vi "pre-processing.vi"() -> ()   [LabVIEW 2015]
uses:
  <vilib>/myRIO/Instrument Drivers/Onboard IO/AudioIn Block/typedefs/AudioIn Block Reference.ctl
  <vilib>/myRIO/Common/Instrument Driver Framework/Utilities/typedefs/myRIO Generic Hardware Reference.ctl
  <vilib>/myRIO/Common/Instrument Driver Framework/Utilities/typedefs/Hardware Version Enum.ctl
  <vilib>/myRIO/Common/Instrument Driver Framework/Utilities/typedefs/myRIO v1.0 Reference.ctl
  <vilib>/myRIO/Common/Instrument Driver Framework/Utilities/typedefs/Generic FPGA Reference.ctl
  <vilib>/myRIO/Common/Instrument Driver Framework/myRIO v1.0/AudioIn Block/typedefs/AudioIn Block Channels List.ctl
  <vilib>/myRIO/Common/Instrument Driver Framework/myRIO v1.0/AudioIn Block/typedefs/AudioIn Block Channels Enum.ctl
  <vilib>/myRIO/Common/Instrument Driver Framework/Utilities/typedefs/Analog Scaling Constants.ctl
  <vilib>/userdefined/High Color/nirio_resource_hc.ctl
  <vilib>/myRIO/Common/Instrument Driver Framework/Utilities/vis/Is FPGA Ref Available.vi
  <vilib>/myRIO/Common/Instrument Driver Framework/myRIO v1.0/AudioIn Block/vis/myRIO v1.1 Open Throughput AudioIn (N Samples).vi
  <vilib>/myRIO/Instrument Drivers/Onboard IO/AudioIn Block/vis/Read.vi
  <vilib>/myRIO/Common/Instrument Driver Framework/Utilities/vis/Validate Channels.vi
  <vilib>/Utility/VariantDataType/GetNumericInfo.vi
  <vilib>/Utility/error.llb/Error Cluster From Error Code.vi
  <vilib>/myRIO/Common/Instrument Driver Framework/myRIO v1.0/myRIO v1.1 Open Throughput.vi
  <vilib>/myRIO/Common/Instrument Driver Framework/myRIO v1.0/AudioIn Block/vis/myRIO v1.0 Get Scaling Constants AudioIn Block.vi
  <vilib>/myRIO/Common/Instrument Driver Framework/myRIO v1.0/AudioIn Block/vis/myRIO v1.0 Reserve AudioIn Block.vi
  <vilib>/myRIO/Common/Instrument Driver Framework/myRIO v1.0/myRIO v1.0 Close.vi
  <vilib>/myRIO/Common/Instrument Driver Framework/myRIO v1.0/AudioIn Block/vis/myRIO v1.0 AudioIn Block Read.vi
  <vilib>/express/express analysis/Spectral/Block/exnSpectralBlock spectral measurements power poly.vi
  <vilib>/express/express analysis/Spectral/Block/exnSpectralBlock spectral measurements power WFM.vi
  <vilib>/measure/matone.llb/Extract Multiple Tone Information 1 Chan.vi
  <vilib>/myRIO/Express VI/Onboard IO/AudioIn/AudioIn Express VI.xnode
  <vilib>/myRIO/Instrument Drivers/Onboard IO/AudioIn Block/vis/myRIO AudioIn N Samples Open.xnode
  <vilib>/express/express analysis/Spectral/XNode/ExpressSpectralMeasurementsBlockNode.xnode
  <vilib>/measure/NI_MAPro.lvlib
  <vilib>/myRIO/Instrument Drivers/Onboard IO/AudioIn Block/AudioIn Block.lvlib
panel:
  out "Numeric 6":dbl
  out "Numeric 5":dbl
  out "Numeric 4":dbl
  out "Numeric 3":dbl
  out "Numeric 2":dbl
  out "Numeric 1":dbl
  out "Waveform Graph":cluster{"f0":dbl, "df":dbl, "magnitude":dbl[]}(graph)
  out "Waveform Chart":dbl[](graph)
  in  "stop":bool
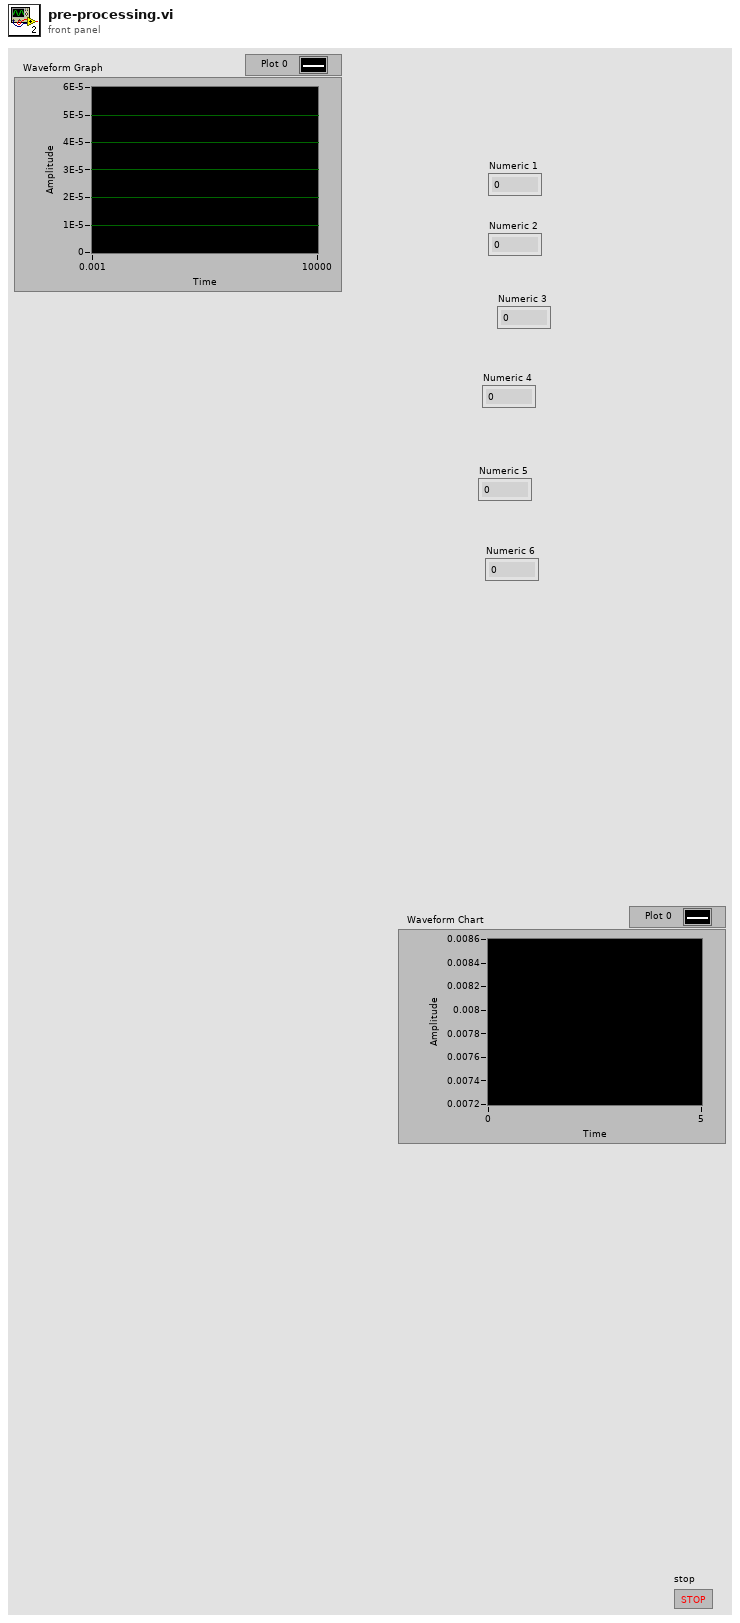
[diagram p1: front panel]
types:
  T1 = cluster{"averaging mode":u16, "weighting mode":u16, "number of averages":u32}
  T2 = cluster{"dB On (F)":bool, "unwrap phase (F)":bool, "convert to degree (F)":bool}
  T3 = typedef "AudioIn Block.lvlib/AudioIn Block Reference.ctl" = cluster{"myRIO Reference":T4, "AudioIn (N Samples) Channels List":T8, "AudioIn (N Samples) Scaling Constants List":T10[]}
  T4 = typedef "myRIO Generic Hardware Reference.ctl" = cluster{"myRIO Model":T5, "myRIO Hardware Reference":T6}
  T5 = typedef "Hardware Version Enum.ctl" = enum16{"Unknown", "myRIO-1900", "myRIO-1950", "roboRIO"}
  T6 = typedef "myRIO v1.0 Reference.ctl" = cluster{"Generic FPGA Reference":T7, "Allow multiple opens":bool}
  T7 = typedef "Generic FPGA Reference.ctl" = refnum<k20>
  T8 = typedef "AudioIn Block Channels List.ctl" = T9[]
  T9 = typedef "AudioIn Block Channels Enum.ctl" = enum16{"Not Connected", "AudioIn/Left (N Samples)", "AudioIn/Right (N Samples)"}
  T10 = typedef "Analog Scaling Constants.ctl" = cluster{"LSB Weight (Volts)":dbl, "Offset (Volts)":dbl, "Signed?":bool}
  T11 = typedef "nirio_resource_hc.ctl" = tag
  T12 = cluster{"detected frequency":dbl, "detected amplitude":dbl, "detected phase (deg)":dbl}[]
  T13 = cluster{"multiple tone information[0]":cluster{"detected frequency":dbl, "detected amplitude":dbl, "detected phase (deg)":dbl}, "multiple tone information[1]":cluster{"detected frequency":dbl, "detected amplitude":dbl, "detected phase (deg)":dbl}, "multiple tone information[2]":cluster{"detected frequency":dbl, "detected amplitude":dbl, "detected phase (deg)":dbl}, "multiple tone information[3]":cluster{"detected frequency":dbl, "detected amplitude":dbl, "detected phase (deg)":dbl}, "multiple tone information[4]":cluster{"detected frequency":dbl, "detected amplitude":dbl, "detected phase (deg)":dbl}, "multiple tone information[5]":cluster{"detected frequency":dbl, "detected amplitude":dbl, "detected phase (deg)":dbl}, "multiple tone information[6]":cluster{"detected frequency":dbl, "detected amplitude":dbl, "detected phase (deg)":dbl}, "multiple tone information[7]":cluster{"detected frequency":dbl, "detected amplitude":dbl, "detected phase (deg)":dbl}, "multiple tone information[8]":cluster{"detected frequency":dbl, "detected amplitude":dbl, "detected phase (deg)":dbl}}
  T14 = cluster{"detected frequency":dbl, "detected amplitude":dbl, "detected phase (deg)":dbl}
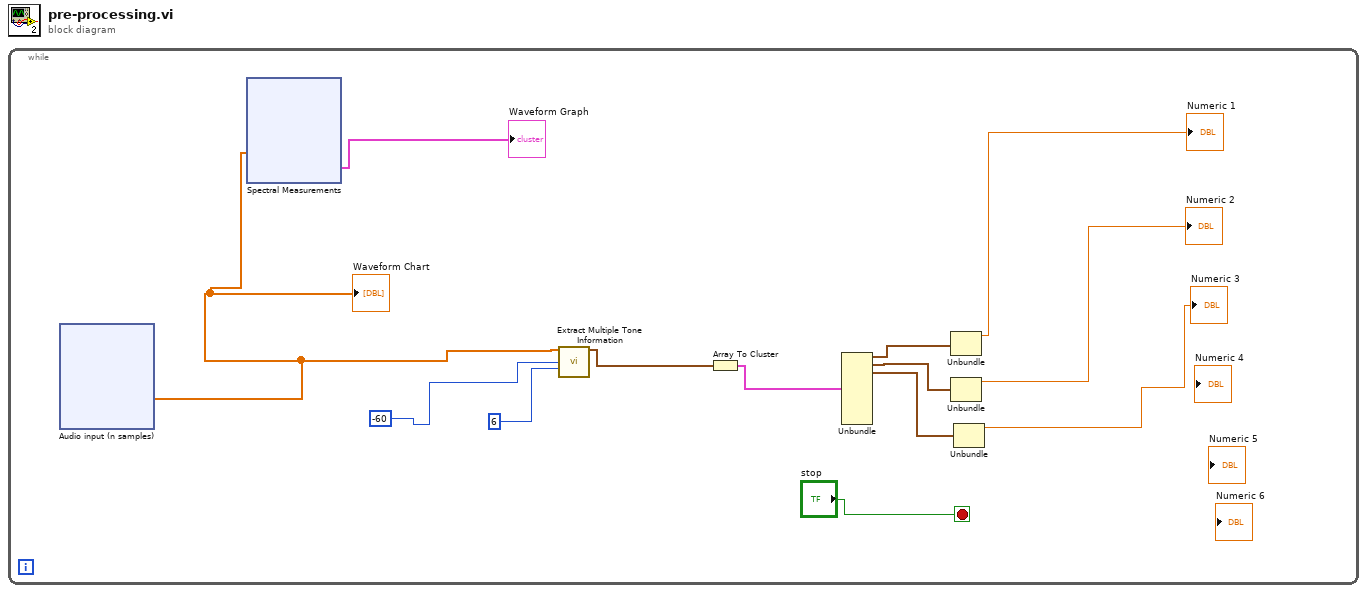
[diagram p0: block diagram]
diagram:
  n1 = while {
    stop <- "stop" stop-if-true
    n2 = xnode "Audio input (n samples)"() -> ("AudioIn/Left (N Samples)"=w5:dbl[])  [unwired: 1 in, 2 out]
    "Waveform Chart" <- w5
    n3 = xnode "Spectral Measurements"("Signals"=w5) -> ("Power Spectrum"=→"Waveform Graph":cluster{"f0":dbl, "df":dbl, "magnitude":dbl[]})  [unwired: 1 in, 1 out]
    n4 = call-poly <vilib>:"Extract Multiple Tone Information.vi"("time signal in"=w5, "threshold"=-60, "max num tones"=6) -> ("multiple tone information"=w11:T12)  [unwired: 10 in, 2 out]
    n5 = Array To Cluster(array=w11) -> (cluster=w10:T13)
    n6 = Unbundle(w10) -> ("multiple tone information[0]"=w9:T14, "multiple tone information[1]"=w8:T14, "multiple tone information[2]"=w7:T14)  [unwired: 6 out]
    n7 = Unbundle(w9) -> ("detected frequency"=→"Numeric 1":dbl)  [unwired: 2 out]
    n8 = Unbundle(w8) -> ("detected frequency"=→"Numeric 2":dbl)  [unwired: 2 out]
    n9 = Unbundle(w7) -> ("detected frequency"=→"Numeric 3":dbl)  [unwired: 2 out]
  }
